vi "EnchantedRoomParamsStack.vi"(8 "error in (no error)":errorcluster, 10 "Spell":refnum<class "Spell.lvclass">, 11 "RoomNumber":i32) -> (0 "error out":errorcluster, 2 "HierarchyParams":variant[](array[variant]), 3 "EnchantedRoom":refnum<class "EnchantedRoom.lvclass">)   [LabVIEW 2020, in "EnchantedRoom.lvclass"]
uses:
  EnchantedRoom.lvclass
  E:/GitHub/Design-Patterns-GoF_-_NI-LV/Creational/GoFcommonClasses/ConcreteMazeSite/Room/Room.lvclass
  Spell/Spell.lvclass
  Room/Protected/property/Read RoomParams.vi
  Protected/property/EnchantedRoomParams.vi
  EnchantedRoom.lvclass/EnchantedRoom.ctl
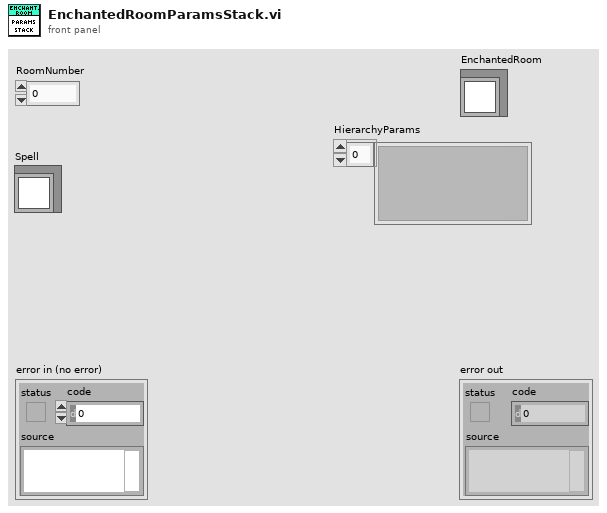
[diagram p1: front panel]
types:
  T1 = typedef "Room.lvclass/RoomParams.ctl" = cluster{"roomNumber":i32}
  T2 = typedef "EnchantedRoom.lvclass/EnchantedRoomParams.ctl" = cluster{"Spell":refnum<class "Spell.lvclass">}
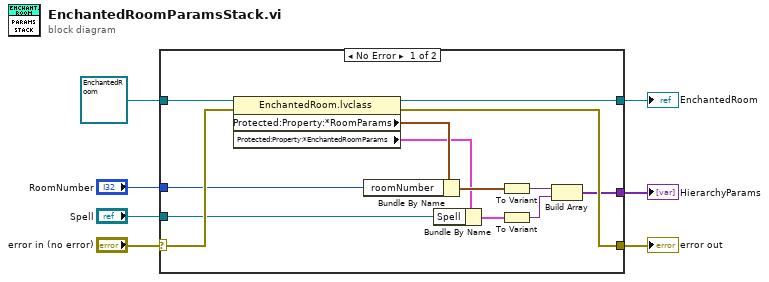
[diagram p0: block diagram]
diagram:
  n1 = case shown="No Error" "error in (no error)" {
    selector: "error in (no error)" -> [w20 w22]
    tunnel: [w17 w22] -> w6
    tunnel: "Spell" -> [w12 _]
    tunnel: refnum<class "EnchantedRoom.lvclass"> refnum ("Milk") -> [w19 w21]
    tunnel: [w18 w21] -> w4
    tunnel: [w16 _] -> w3
    tunnel: "RoomNumber" -> [w10 _]
    frame No Error {
      n2 = property class="EnchantedRoom.lvclass"(reference=w19, error in=w20) -> (reference out=w18:refnum<class "EnchantedRoom.lvclass">, error out=w17:errorcluster, "Protected:Property:*RoomParams"=w13:T1, "Protected:Property:*EnchantedRoomParams"=w11:T2)
      n3 = Bundle By Name(cluster=w13, "roomNumber"=w10) -> (w15:T1)
      n4 = Bundle By Name(cluster=w11, "Spell"=w12) -> (w8:T2)
      n5 = To Variant(anything=w15) -> (Variant=w14:variant)
      n6 = To Variant(anything=w8) -> (Variant=w9:variant)
      n7 = Build Array(w14, w9) -> (w16:variant[])
    }
    frame Error {
    }
  }
  "error out" <- w6
  "EnchantedRoom" <- w4
  "HierarchyParams" <- w3
